vi "bitpacked_bitarray_to_counts.vi"(11 "Bit Array":bool[](array[boolean])) -> (3 "Integer Array":i16[](array[numeric]))   [LabVIEW 2014]
doc: "Seperates out 12 bit samples and converts them to 16bit unsigned integers."
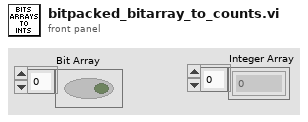
[diagram p1: front panel]
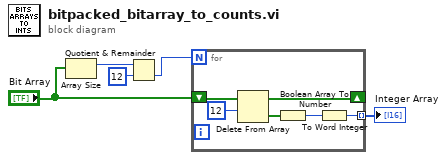
[diagram p0: block diagram]
diagram:
  n1 = Array Size(array="Bit Array") -> (size(s)=w2:i32)
  n2 = Quotient & Remainder(x=w2, y=12) -> (floor(x/y)=w4:i32)  [unwired: 1 out]
  n3 = for {
    N: w4 -> [_]
    shift-right: [w9] -> _
    shift-left: "Bit Array" -> [w11]
    tunnel: [w7] -> w1 mode=indexing
    n4 = Delete From Array(array=w11, length=12) -> (deleted portion=w8:bool[], array with subset deleted=w9:bool[])  [unwired: 1 in]
    n5 = Boolean Array To Number(Boolean array=w8) -> (number=w6:u32)
    n6 = To Word Integer(number=w6) -> (16bit integer=w7:i16)
  }
  "Integer Array" <- w1
